vi "Create Notifiers.vi"(8 "error in":errorcluster) -> (0 "error out":errorcluster, 3 "Notifiers":T1)   [LabVIEW 2017]
uses:
  Notifiers.ctl
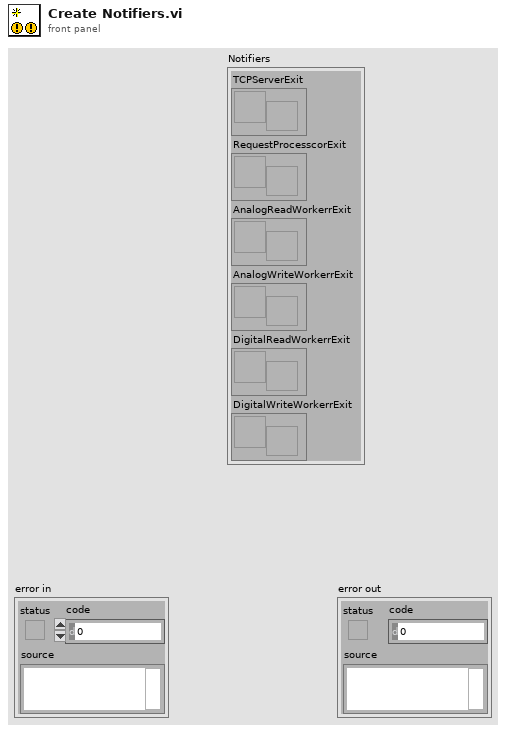
[diagram p1: front panel]
types:
  T1 = typedef "Notifiers.ctl" = cluster{"TCPServerExit":refnum<notifier>, "RequestProcesscorExit":refnum<notifier>, "AnalogReadWorkerrExit":refnum<notifier>, "AnalogWriteWorkerrExit":refnum<notifier>, "DigitalReadWorkerrExit":refnum<notifier>, "DigitalWriteWorkerrExit":refnum<notifier>}
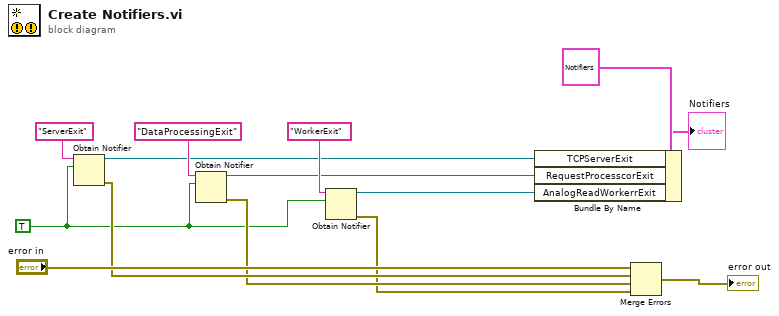
[diagram p0: block diagram]
diagram:
  w6 = TRUE
  n1 = Obtain Notifier(name (unnamed)="ServerExit", notification data type=w6) -> (notifier out=w3:refnum<notifier>, error out=w9:errorcluster)  [unwired: 2 in, 1 out]
  n2 = Obtain Notifier(name (unnamed)="DataProcessingExit", notification data type=w6) -> (notifier out=w2:refnum<notifier>, error out=w8:errorcluster)  [unwired: 2 in, 1 out]
  n3 = Obtain Notifier(name (unnamed)="WorkerExit", notification data type=w6) -> (notifier out=w1:refnum<notifier>, error out=w7:errorcluster)  [unwired: 2 in, 1 out]
  n4 = Bundle By Name(cluster=T1 {"TCPServerExit"=refnum, "RequestProcesscorExit"=refnum, "AnalogReadWorkerrExit"=refnum, "AnalogWriteWorkerrExit"=refnum, "DigitalReadWorkerrExit"=refnum, "DigitalWriteWorkerrExit"=refnum} ("Notifiers"), "TCPServerExit"=w3, "RequestProcesscorExit"=w2, "AnalogReadWorkerrExit"=w1) -> (→"Notifiers":T1)
  n5 = Merge Errors("error in", w9, w8, w7) -> (→"error out":errorcluster)
